vi "Conf COM.vi"(8 "error in (no error)":errorcluster, 11 "Conection Data In":T1) -> (0 "error out":errorcluster, 3 "Conection Data Out":T1)   [LabVIEW 2014, in "SJ-210.lvlib" / "SJ-210.lvclass"]
uses:
  SJ-210Class/SJ-210.lvclass
  API/Typedef/Connection Data.ctl
  API/SJ-210 Lib.lvlib
panel:
  in  "Save Button":bool=TRUE
  # "Seleccionar Puerto"
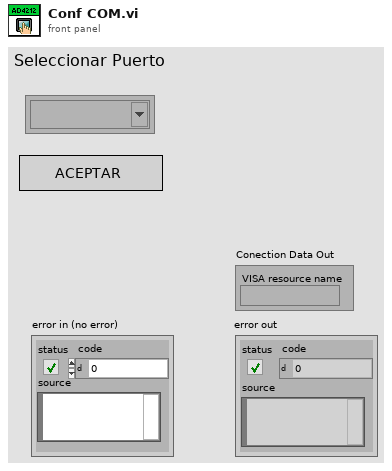
[diagram p1: front panel]
types:
  T1 = typedef "SJ-210 Lib.lvlib/Connection Data.ctl" = cluster{"VISA resource name":refnum<visa-resource-name>}
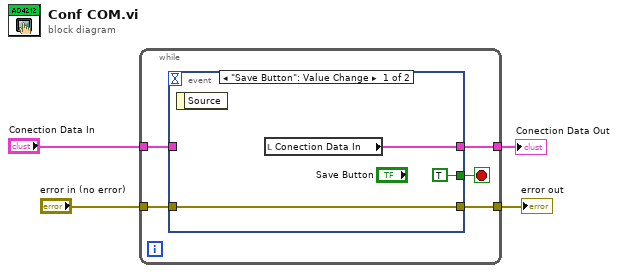
[diagram p0: block diagram]
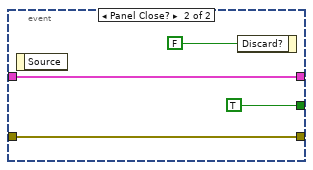
[diagram p2: hidden frame]
diagram:
  n1 = while {
    tunnel: [w8] -> w4
    tunnel: "error in (no error)" -> [w7]
    tunnel: "Conection Data In" -> [w6]
    tunnel: [w5] -> w1
    stop <- w9 stop-if-true
    n2 = event shown="[0] \"Save Button\": Value Change" {
      selector: _ -> [_ _]
      dyn-events: _ -> [_ _]
      timeout: _ -> [_ _]
      tunnel: [TRUE ("Save Button") TRUE ("Save Button")] -> w9
      tunnel: [w12 w14] -> w8
      tunnel: w7 -> [w12 w14]
      tunnel: w6 -> [_ w13]
      tunnel: [w11 w13] -> w5
      event "Save Button": Value Change {
        n3 = event-data() -> ()  [unwired: 1 in, 1 out]
        n4 = local read "Conection Data In"() -> (w11:T1)
      }
      event Panel Close? {
        n5 = event-data() -> ()  [unwired: 1 in, 1 out]
        n6 = event-data("Discard?"=FALSE) -> ()  [unwired: 1 in, 1 out]
      }
    }
  }
  "error out" <- w4
  "Conection Data Out" <- w1
